vi "Picture Prompt_Typical_Calibration.vi"(8 "error in (no error)":errorcluster) -> (0 "error out":errorcluster, 2 "OK Button Pressed?":bool)   [LabVIEW 2015]
panel:
  in  "OK Button":bool
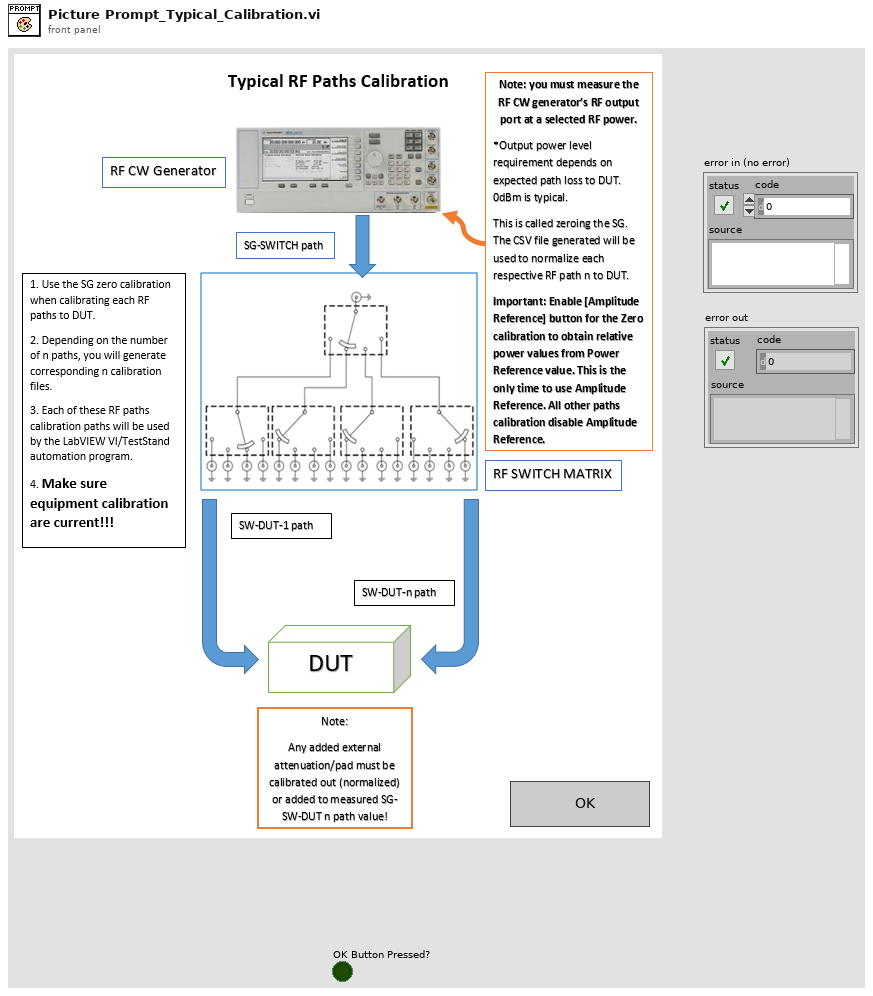
[diagram p1: front panel]
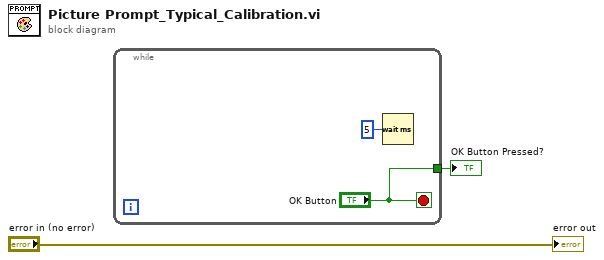
[diagram p0: block diagram]
diagram:
  n1 = while {
    tunnel: ["OK Button"] -> w1
    stop <- "OK Button" stop-if-true
    n2 = Wait (ms)(milliseconds to wait=u32 5) -> ()  [unwired: 1 out]
  }
  "OK Button Pressed?" <- w1
  "error out" <- "error in (no error)"
